vi "Gauss-Seidel Iteration (abs residual).vi"(4 "max. iters":i32=10000, 5 "res. tol":dbl=1e-05, 6 "B":dbl[](array[numeric])=[6.0, 25.0, -11.0, 15.0], 7 "A":dbl[][](array[numeric])=[[10.0, -1.0, 2.0, 0.0], [-1.0, 11.0, -1.0, 3.0], [2.0, -1.0, 10.0, -1.0], [0.0, 3.0, -1.0, 8.0]]) -> (0 "Converged?":bool=TRUE, 1 "Iterations":i32=10, 3 "X":dbl[](array[numeric])=[1.0, 2.0, -1.0, 1.0])   [LabVIEW 2017]
uses:
  <vilib>/Analysis/baseanly.llb/A x Vector.vi
  <vilib>/Analysis/NI_AALBase.lvlib
panel:
  in  "Stop":bool
  out "Residual":sgl(graph)
  # "PN 21/10/17"
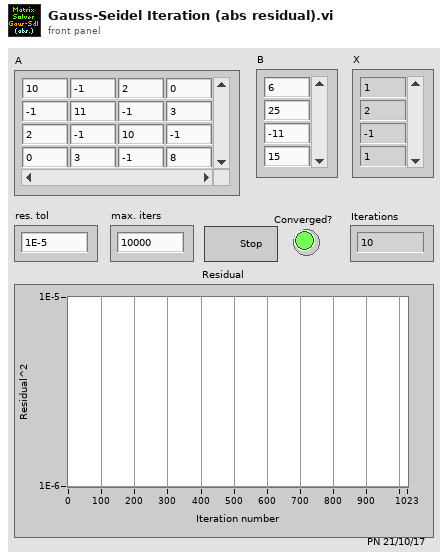
[diagram p1: front panel]
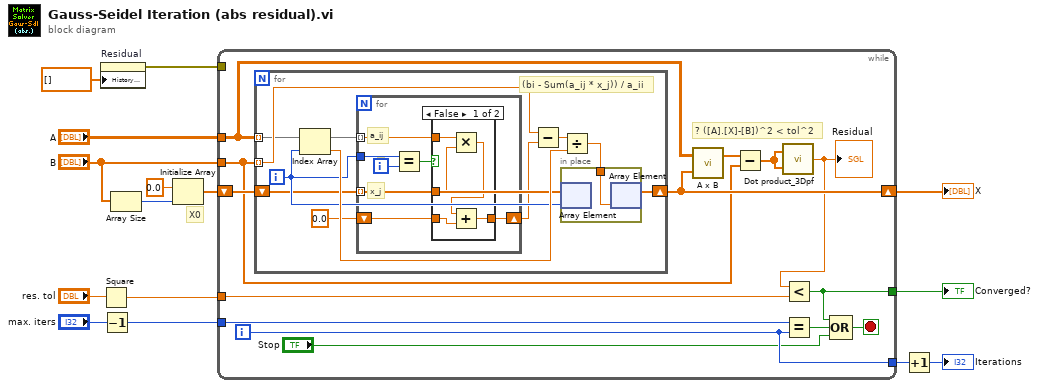
[diagram p0: block diagram]
diagram:
  # "X0"
  n1 = property on="Residual" class="WFChart (strict)"("History Data"=sgl[] []) -> (error out=w3:errorcluster)  [unwired: 2 in, 1 out]
  n2 = Square(x="res. tol") -> (x^2=w2:dbl)
  n3 = Decrement(x="max. iters") -> (x-1=w10:i32)
  n4 = Array Size(array="B") -> (size(s)=w14:i32)
  n5 = Initialize Array(0.0 ("element"), w14) -> (w13:dbl[])
  n6 = while {
    tunnel: "A" -> [w24]
    tunnel: "B" -> [w19]
    tunnel: w2 -> [w29]
    shift-right: [w23] -> w6
    shift-left: w13 -> [w21]
    tunnel: w10 -> [w27]
    tunnel: [w26] -> w9
    tunnel: w3 -> [_]
    tunnel: [w17] -> w1
    i -> [w26]
    stop <- w28 stop-if-true
    # "? ([A].[X]-[B])^2 < tol^2"
    n7 = for {
      tunnel: w19 -> [w39] mode=indexing
      tunnel: w24 -> [w36] mode=indexing
      shift-right: [w32] -> w23
      shift-left: w21 -> [w34]
      i -> [w35]
      # "(bi - Sum(a_ij * x_j)) / a_ii"
      n8 = Index Array(array=w36, index=w35) -> (element=w37:dbl)
      n9 = for {
        tunnel: w35 -> [w46]
        tunnel: w36 -> [w44] mode=indexing
        tunnel: w34 -> [w43] mode=indexing
        shift-right: [w42] -> w30
        shift-left: 0.0 ("element") -> [w41]
        i -> [w47]
        # "x_j"
        # "a_ij"
        # "j"
        n10 = Equal?(x=w46, y=w47) -> (x = y?=w45:bool)
        n11 = case shown="False" w45 {
          tunnel: w44 -> [w52 _]
          tunnel: w43 -> [w51 _]
          tunnel: [w50 w53] -> w42
          tunnel: w41 -> [w49 w53]
          frame False {
            n12 = Multiply(x=w52, y=w51) -> (x*y=w48:dbl)
            n13 = Add(x=w48, y=w49) -> (x+y=w50:dbl)
          }
          frame True {
          }
        }
      }
      n14 = Subtract(x=w39, y=w30) -> (x-y=w38:dbl)
      n15 = Divide(x=w38, y=w37) -> (x/y=w33:dbl)
      n16 = in-place {
        in-place-border: w33 -> [w40]
        n17 = in-place-array #1(w34, w35) -> ()  [unwired: 1 out]
        n18 = in-place-array #1(w40) -> (w32:dbl[])  [unwired: 1 out]
      }
    }
    n19 = call-poly <vilib>:"A x B.vi"("Vector"=w23, "A"=w24) -> ("A x Vector"=w22:dbl[])  [unwired: 1 out]
    n20 = Subtract(x=w22, y=w19) -> (x-y=w25:dbl[])
    n21 = call "Dot product_3Dpf.vi"("B"=w25, "A"=w25) -> ("A . B"=w20:sgl)
    "Residual" <- w20
    n22 = Less?(x=w20, y=w29) -> (x < y?=w17:bool)
    n23 = Equal?(x=w27, y=w26) -> (x = y?=w18:bool)
    n24 = Compound Arithmetic op=OR(w17, w18, "Stop") -> (w28:bool)
  }
  "X" <- w6
  "Converged?" <- w1
  n25 = Increment(x=w9) -> (x+1=→"Iterations":i32)
